vi "Peek at model queue.vi"(8 "error in (no error)":errorcluster, 11 "Check for specific pending state (don't check)":string) -> (0 "error out":errorcluster, 1 "At least one state pending":bool, 2 "States waiting to run":i32, 3 "Specific pending state found":bool)   [LabVIEW 2018]
doc: "Looks ahead at the queue for the Model to see if there are pending actions after the current one.\n\nOptionally, the queue can be checked to see if a specific action is pending (for instance, checking to see if a Cancel action was queued up) and this outputs a True boolean if there is one waiting."
uses:
  <vilib>/Utility/error.llb/Trim Whitespace.vi
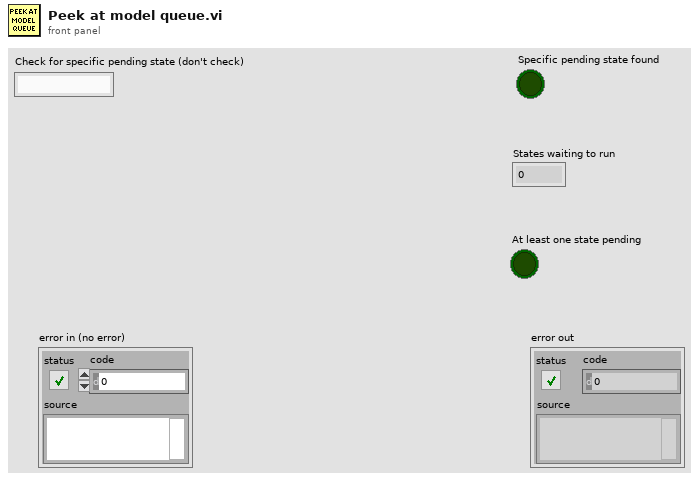
[diagram p1: front panel]
types:
  T1 = typedef "Model queue data.ctl" = cluster{"State":string, "Data":variant, "Next state if error":string}
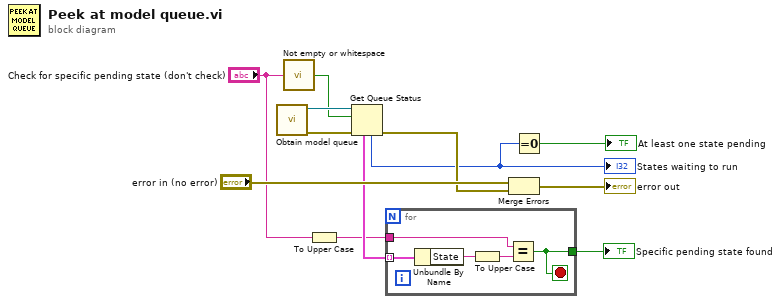
[diagram p0: block diagram]
diagram:
  n1 = call "Obtain model queue.vi"() -> ("error out"=w10:errorcluster, "Model loop queue"=w9:refnum<queue>)  [unwired: 10 in]
  n2 = call <userlib>:"Not empty or whitespace.vi"("String"="Check for specific pending state (don't check)") -> ("Not empty or all whitespace"=w8:bool)  [unwired: 4 in]
  n3 = To Upper Case(1:"Check for specific pending state (don't check)") -> (0:w2:string)
  n4 = Get Queue Status(queue=w9, return elements? (F)=w8, error in (no error)=w10) -> (error out=w7:errorcluster, # elements in queue=w6:i32, elements=w4:T1[])  [unwired: 5 out]
  "States waiting to run" <- w6
  n5 = for {
    tunnel: w4 -> [w17] mode=indexing
    tunnel: w2 -> [w14]
    tunnel: [w13] -> w1
    stop <- w13 stop-if-true
    n6 = Unbundle By Name(w17) -> ("State"=w16:string)
    n7 = To Upper Case(1:w16) -> (0:w15:string)
    n8 = Equal?(x=w14, y=w15) -> (x = y?=w13:bool)
  }
  "Specific pending state found" <- w1
  n9 = Merge Errors("error in (no error)", w7) -> (→"error out":errorcluster)
  n10 = Equal To 0?(x=w6) -> (x = 0?=→"At least one state pending":bool)
